vi "Dual Channel Temperature Log with Headers.vi"() -> ()   [LabVIEW 2012]
doc: "This VI acquires temperature values every second and maintains a running average of the last five temperature measurements. This VI displays and logs both the raw data and the running average."
panel:
  in  "Stop Button":bool
  out "Temperature History":cluster{dbl, "Temperature Value":dbl}(graph)
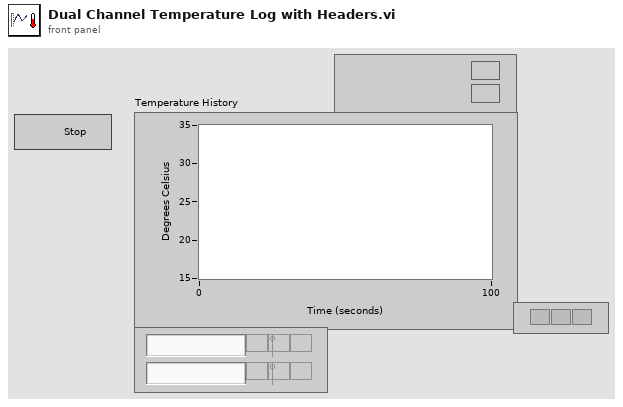
[diagram p1: front panel]
types:
  T1 = enum16{"open", "replace", "create", "open or create", "replace or create", "replace or create with confirmation"}
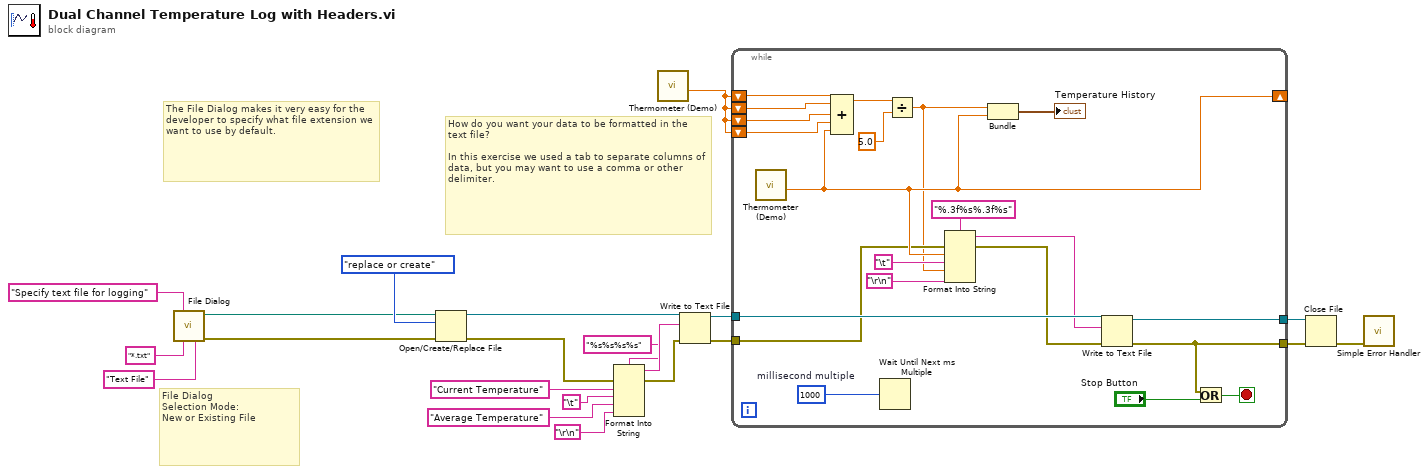
[diagram p0: block diagram]
diagram:
  # "How do you want your data to be formatted in the text file? \n\nIn this exercise we used a tab to separate columns of data, but you may want to use a comma or other delimiter."
  # "File Dialog \nSelection Mode:\nNew or Existing File"
  # "The File Dialog makes it very easy for the developer to specify what file extension we want to use by default."
  n1 = call "File Dialog"("prompt"="Specify text file for logging" ("pattern label"), "pattern (all files)"="*.txt", "pattern label"="Text File") -> ("selected path"=w15:path, "error out"=w2:errorcluster)  [unwired: 9 in, 2 out]
  n2 = Open/Create/Replace File(file path (use dialog)=w15, error in=w2, operation (0:open)=T1."replace or create") -> (refnum out=w16:refnum<file>, error out=w4:errorcluster)  [unwired: 4 out]
  n3 = Format Into String(format string="%s%s%s%s", error in=w4, "Current Temperature" ("string"), "\t", "Average Temperature" ("string"), "\r\n" ("End of Line Constant")) -> (resulting string=w5:string, error out=w3:errorcluster)  [unwired: 1 in]
  n4 = call "Thermometer (Demo).vi"() -> ("Temperature Value"=w21:dbl)  [unwired: 11 in]
  n5 = Write to Text File(file (use dialog)=w16, text=w5, error in=w3) -> (refnum out=w12:refnum<file>, error out=w11:errorcluster)  [unwired: 2 out]
  n6 = while {
    shift-right: [w29] -> _
    shift-left: w21 -> [w41]
    shift-left: w21 -> [w40]
    shift-left: w21 -> [w37]
    shift-left: w21 -> [w36]
    tunnel: w11 -> [w27]
    tunnel: [w32] -> w19
    tunnel: w12 -> [w34]
    tunnel: [w33] -> w18
    stop <- w30 stop-if-true
    w42 = u32 1000  # millisecond multiple
    n7 = call "Thermometer (Demo).vi"() -> ("Temperature Value"=w29:dbl)  [unwired: 11 in]
    n8 = Compound Arithmetic op=ADD(w41, w40, w37, w36, w29) -> (w39:dbl)
    n9 = Wait Until Next ms Multiple(millisecond multiple=w42) -> ()  [unwired: 1 out]
    n10 = Divide(x=w39, y=5.0) -> (x/y=w23:dbl)
    n11 = Format Into String "Format Into String"(format string="%.3f%s%.3f%s", error in=w27, w29, "\t", w23, "\r\n") -> (resulting string=w28:string, error out=w26:errorcluster)  [unwired: 1 in]
    n12 = Bundle(w23, "Temperature Value"=w29) -> (→"Temperature History":cluster{dbl, "Temperature Value":dbl})  [unwired: 1 in]
    n13 = Write to Text File(file (use dialog)=w34, text=w28, error in=w26) -> (refnum out=w33:refnum<file>, error out=w32:errorcluster)  [unwired: 2 out]
    n14 = Or(x=w32, y="Stop Button") -> (x .or. y?=w30:bool)
  }
  n15 = Close File(refnum=w18, error in=w19) -> (error out=w20:errorcluster)  [unwired: 1 out]
  n16 = call <vilib>:"Simple Error Handler.vi"("error in (no error)"=w20) -> ()  [unwired: 1 in, 8 out]
